vi "LT_unbundle_values.vi"(11 "Status values":T1) -> (0 "volt":dbl, 1 "current":dbl, 2 "temp":u16, 3 "freq":u16)   [LabVIEW 2019]
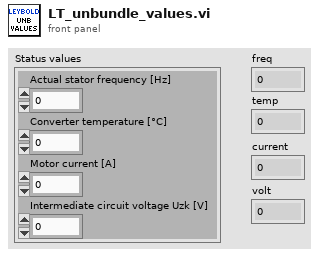
[diagram p1: front panel]
types:
  T1 = cluster{"Actual stator frequency [Hz]":u16, "Converter temperature [°C]":u16, "Motor current [A]":dbl, "Intermediate circuit voltage Uzk [V]":dbl}
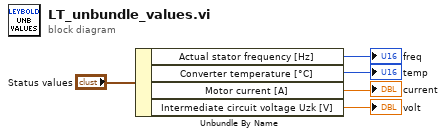
[diagram p0: block diagram]
diagram:
  n1 = Unbundle By Name("Status values") -> ("Actual stator frequency [Hz]"=→"freq":u16, "Converter temperature [°C]"=→"temp":u16, "Motor current [A]"=→"current":dbl, "Intermediate circuit voltage Uzk [V]"=→"volt":dbl)
